vi "DimIndicators.dic_release_service.vi"(0 "controlRef":refnum<vi>, 5 "error in (no error)":errorcluster) -> (19 "error out":errorcluster)   [LabVIEW 2015, in "DimIndicators.lvlib"]
doc: "Unregisters a control from a DIM service."
uses:
  DimIndicators.lvlib
  DimIndicators.actionType.ctl
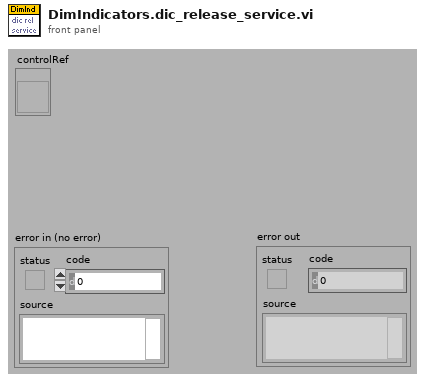
[diagram p1: front panel]
types:
  T1 = typedef "DimIndicators.lvlib/DimIndicators.actionType.ctl" = enum16{"dic_info_service", "dic_release_service", "init", "getControlRef", "getCallbackID", "close"}
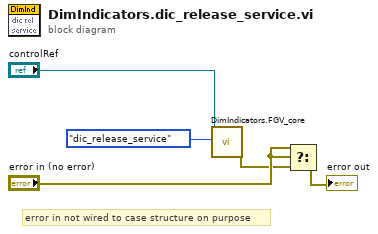
[diagram p0: block diagram]
diagram:
  # "error in not wired to case structure on purpose"
  n1 = call "DimIndicators.FGV_core.vi"("controlRef"="controlRef", "actions"=DimIndicators.actionType."dic_release_service") -> ("error out"=w3:errorcluster)  [unwired: 14 in, 3 out]
  n2 = Select(t="error in (no error)", s="error in (no error)", f=w3) -> (s? t:f=→"error out":errorcluster)
